vi "ex6-2.vi"   [LabVIEW 2013]
uses:
  <vilib>/NXT/Dual Mode Library/Waits/Wait_Num.vi
  <vilib>/NXT/Dual Mode Library/Sensors/EV3_Color_Reflect.vi
  <vilib>/NXT/Dual Mode Library/Display/drawNumber_float.vi
  <vilib>/NXT/NXTIO Xnodes/NXTIONodeSubVIs/LEGOMoveAllMotors.vi
  <vilib>/NXT/Subs/LVHSConnector.ctl
  <vilib>/NXT/NXTIO Xnodes/NXTIOXNode/NXTIO.xnode
  <vilib>/NXT/LegoClasses/BrickReference/BrickReference.lvclass
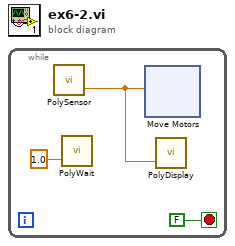
[diagram p0: block diagram]
diagram:
  n1 = while {
    stop <- FALSE stop-if-true
    n2 = call-poly <vilib>:"PolySensor.vi"() -> ("Scaled Value"=w1:sgl)  [unwired: 3 in, 1 out]
    n3 = call-poly <vilib>:"PolyWait.vi"("Time (1 sec)"=sgl 1.0) -> ()  [unwired: 3 in, 1 out]
    n4 = xnode "Move Motors"("Power/Speed 1"=w1) -> ()  [unwired: 2 in, 1 out]
    n5 = call-poly <vilib>:"PolyDisplay.vi"("number"=w1) -> ()  [unwired: 3 in, 1 out]
  }
